vi "Write Overlay colors.vi"(8 "error in (no error)":errorcluster, 10 "Overlay colors":cluster{"Border":u32, "Text":u32}={"Border"=16448250, "Text"=16448250}, 11 "Overlay Base in":refnum<class "Analyze Compound Results Base.lvclass">) -> (0 "error out":errorcluster, 3 "Overlay Base out":refnum<class "Analyze Compound Results Base.lvclass">)   [LabVIEW 2014, in "Analyze Compound Results Base.lvclass"]
uses:
  Analyze Compound Results Base.lvclass
  Analyze Compound Results Base.lvclass/Analyze Compound Results Base.ctl
  Results Base/Analyze Results Base.lvclass
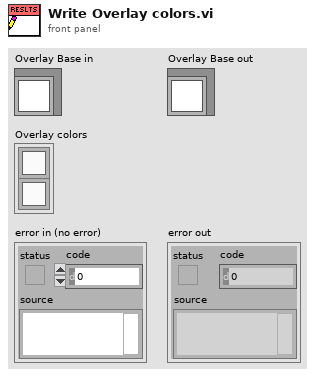
[diagram p1: front panel]
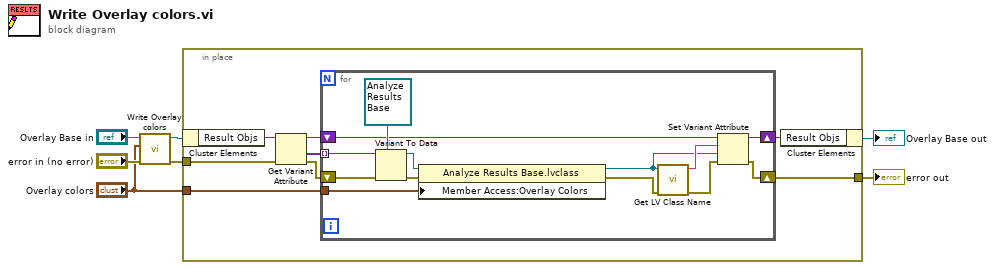
[diagram p0: block diagram]
diagram:
  n1 = call-parent "Write Overlay colors.vi"("error in (no error)"="error in (no error)", "Overlay colors"="Overlay colors", "Overlay Base in"="Overlay Base in") -> ("error out"=w4:errorcluster, "Overlay Base out"=w5:refnum<class "Analyze Compound Results Base.lvclass">)  [unwired: 7 in]
  n2 = in-place {
    in-place-border: w4 -> [w9]
    in-place-border: [w13] -> w1
    in-place-border: "Overlay colors" -> [w11]
    n3 = in-place-cluster #1(w5) -> ("Result Objs"=w15:variant)
    n4 = Get Variant Attribute(Variant=w15, error in=w9) -> (duplicate Variant=w12:variant, values=w14:variant[], error out=w8:errorcluster)  [unwired: 2 in, 1 out]
    n5 = for {
      tunnel: w14 -> [w28] mode=indexing
      shift-right: [w21] -> w13
      shift-left: w8 -> [w26]
      shift-right: [w24] -> w10
      shift-left: w12 -> [w25]
      tunnel: w11 -> [w19]
      n6 = Variant To Data(error in=w26, type=refnum<class "Analyze Results Base.lvclass"> refnum ("Analyze Results Base.lvclass"), Variant=w28) -> (data=w23:refnum<class "Analyze Results Base.lvclass">, error out=w17:errorcluster)
      n7 = property class="Analyze Results Base.lvclass"(reference=w23, error in=w17, "Member Access:Overlay Colors"=w19) -> (reference out=w16:refnum<class "Analyze Results Base.lvclass">, error out=w18:errorcluster)
      n8 = call <vilib>:"Get LV Class Name.vi"("error in (no error)"=w18, "object"=w16) -> ("error out"=w22:errorcluster, "class name"=w20:string)  [unwired: 8 in]
      n9 = Set Variant Attribute(Variant=w25, name=w20, value=w16, error in=w22) -> (Variant out=w24:variant, error out=w21:errorcluster)  [unwired: 1 out]
    }
    n10 = in-place-cluster #1("Result Objs"=w10) -> (→"Overlay Base out":refnum<class "Analyze Compound Results Base.lvclass">)
  }
  "error out" <- w1
